vi "sensor cmd config check.vi"(10 "is_valid":string, 11 "device_handle":u32) -> (1 "function return":i32, 2 "is_valid out":string, 3 "device_handle out":u32)   [LabVIEW 2019, in "apdm.lvlib"]
doc: "APDM_EXPORT int apdm_sensor_cmd_config_check(apdm_device_handle_t device_handle, uint8_t *is_valid);"
uses:
  apdm.lvlib
  Lee Lab/CP FES Walking 2018/Code/Working/LabVIEW/apdm.dll
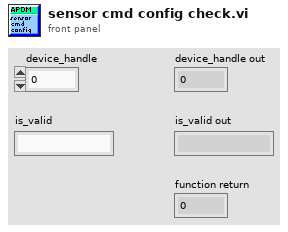
[diagram p1: front panel]
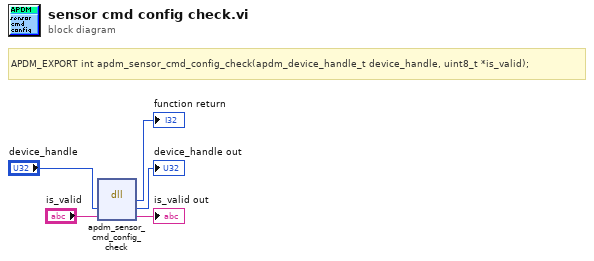
[diagram p0: block diagram]
diagram:
  # "APDM_EXPORT int apdm_sensor_cmd_config_check(apdm_device_handle_t device_handle, uint8_t *is_valid);"
  n1 = dll-call lib="C:/Users/jfalesi/Dropbox/Lee Lab/CP FES Walking 2018/Code/Working/LabVIEW/apdm.*" fn="apdm_sensor_cmd_config_check"("device_handle"="device_handle", "is_valid"="is_valid") -> (→"function return":i32, "device_handle"=→"device_handle out":u32, "is_valid"=→"is_valid out":string)  [unwired: 3 in, 2 out]
